vi "Byte Array Checksum.vi"   [LabVIEW 2020, in "NI_Message Digest API.lvlib"]
doc: "Computes the message digest on a byte array. You must manually select the polymorphic instance you want to use."
uses:
  <vilib>/security/Message Digest/API/NI_Message Digest API.lvlib
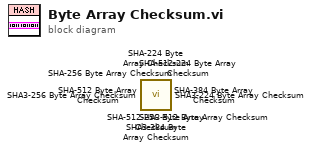
[diagram p0: block diagram]
diagram:
  n1 = call <vilib>:"SHA-512-256 Byte Array Checksum.vi"() -> ()  [unwired: 11 in, 1 out]
  n2 = call <vilib>:"SHA-512-224 Byte Array Checksum.vi"() -> ()  [unwired: 11 in, 1 out]
  n3 = call <vilib>:"SHA-512 Byte Array Checksum.vi"() -> ()  [unwired: 11 in, 1 out]
  n4 = call <vilib>:"SHA-384 Byte Array Checksum.vi"() -> ()  [unwired: 11 in, 1 out]
  n5 = call <vilib>:"SHA-256 Byte Array Checksum.vi"() -> ()  [unwired: 11 in, 1 out]
  n6 = call <vilib>:"SHA-224 Byte Array Checksum.vi"() -> ()  [unwired: 11 in, 1 out]
  n7 = call <vilib>:"SHA3-512 Byte Array Checksum.vi"() -> ()  [unwired: 11 in, 1 out]
  n8 = call <vilib>:"SHA3-384 Byte Array Checksum.vi"() -> ()  [unwired: 11 in, 1 out]
  n9 = call <vilib>:"SHA3-256 Byte Array Checksum.vi"() -> ()  [unwired: 11 in, 1 out]
  n10 = call <vilib>:"SHA3-224 Byte Array Checksum.vi"() -> ()  [unwired: 11 in, 1 out]
